vi "RSZVB Configure Trigger External.vi"(8 "error in (no error)":errorcluster {"code" format="%.0x"}, 9 "Trigger On (0: Falling Edge)":i32(ring) items=["Falling Edge", "Rising Edge"], 10 "Channel (1)":i32=1, 11 "VISA session":refnum<visa-resource-name>) -> (0 "error out":errorcluster {"code" format="%.0x"}, 3 "dup VISA session":refnum<visa-resource-name>)   [LabVIEW 2011]
doc: "This VI configures the external trigger mode. In External trigger mode the measurement is triggered by a low-voltage (3.3 V) external TTL signal applied either to the BNC connector EXT TRIGGER or to pin 2 of the USER CONTROL connector at the rear panel. The two trigger inputs are equivalent; nor additional setting for signal routing is required. \n\nRemote-control command(s):\nTRIGger<Ch>[:SEQuence]:SOURce EXTernal\nTRIGger<Ch>[:SEQuence]:SLOPe POSitive | NEGative"
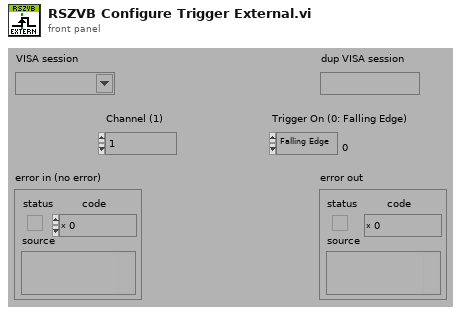
[diagram p1: front panel]
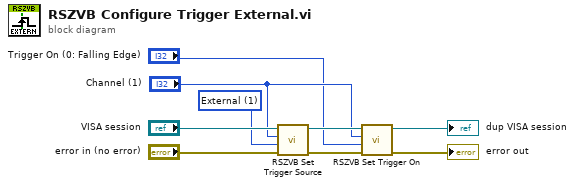
[diagram p0: block diagram]
diagram:
  w7 = 1 items=["Free Run", "External", "Periodic", "Manual", "RF Power"] ("Trigger Source (0: Free Run)")
  n1 = call "RSZVB Set Trigger Source.vi"("error in (no error)"="error in (no error)", "Trigger Source (0: Free Run)"=w7, "Channel (1)"="Channel (1)", "VISA session"="VISA session") -> ("error out"=w5:errorcluster, "dup VISA session"=w6:refnum<visa-resource-name>)  [unwired: 6 in]
  n2 = call "RSZVB Set Trigger On.vi"("error in (no error)"=w5, "Trigger On (0: Falling Edge)"="Trigger On (0: Falling Edge)", "Channel (1)"="Channel (1)", "VISA session"=w6) -> ("error out"=→"error out":errorcluster, "dup VISA session"=→"dup VISA session":refnum<visa-resource-name>)  [unwired: 6 in]
